vi "Maint_Glue_Wind.vi"(0 "VISA Refnum in":refnum<visa-resource-name>, 7 "VISA Refnum in 2":refnum<visa-resource-name>, 11 "error in (no error)":errorcluster) -> (4 "VISA Refnum out":refnum<visa-resource-name>, 8 "VISA Refnum out 2":refnum<visa-resource-name>, 15 "error out":errorcluster)   [LabVIEW 2016]
panel:
  in  "Home Button":bool
  in  "Down Button 2":bool
  in  "Up Button":bool
  in  "error in (no error) 2":errorcluster
  out "error out 2":errorcluster
  in  "Wind Forward":bool
  in  "Wind Reverse":bool
  in  "Glue Down Button":bool
  in  "GLUE UP":bool
  in  "EXIT":bool
  # "GLUE MOTOR"
  # "WIND MOTOR"
  # "STEPPER MOTOR"
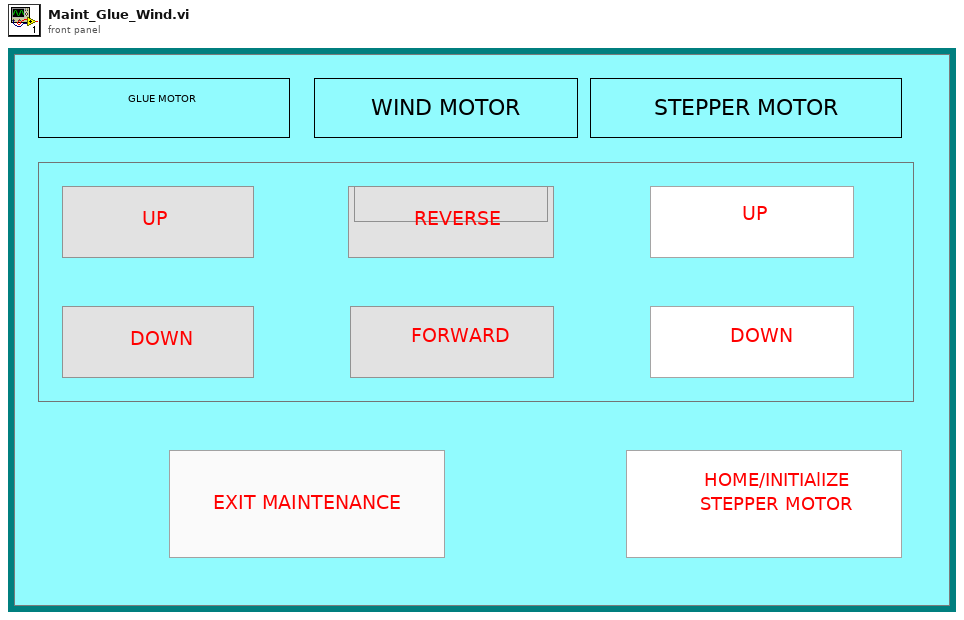
[diagram p1: front panel]
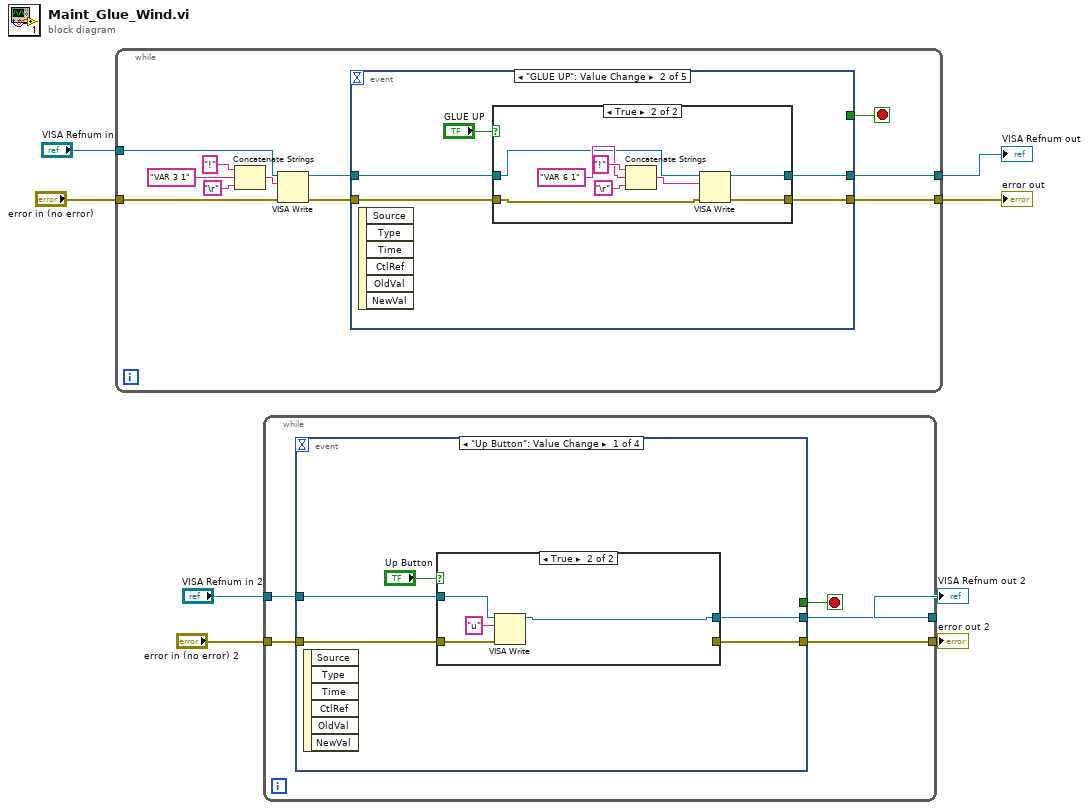
[diagram p0: block diagram]
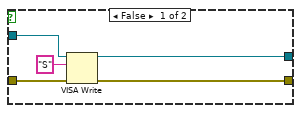
[diagram p2: hidden frame]
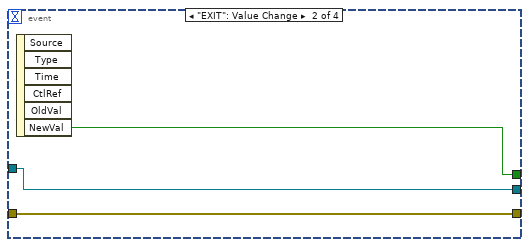
[diagram p3: hidden frame]
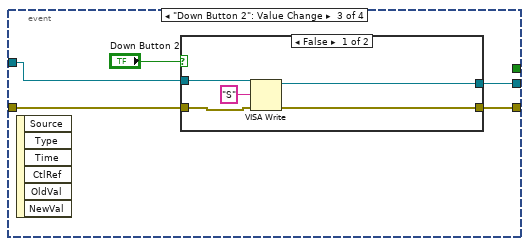
[diagram p4: hidden frame]
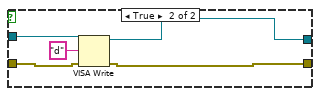
[diagram p5: hidden frame]
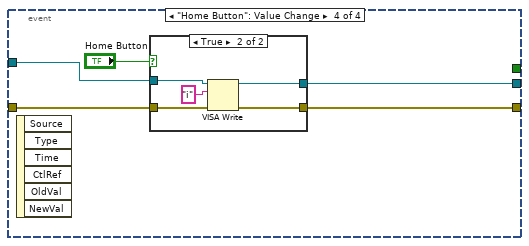
[diagram p6: hidden frame]
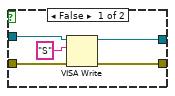
[diagram p7: hidden frame]
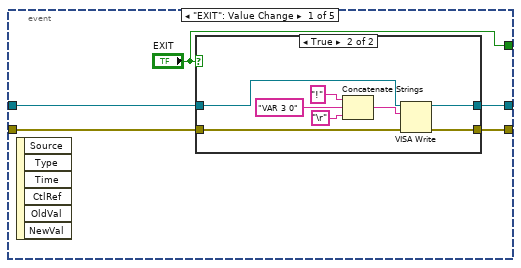
[diagram p8: hidden frame]
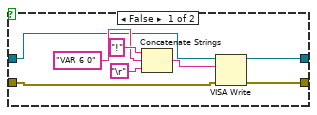
[diagram p10: hidden frame]
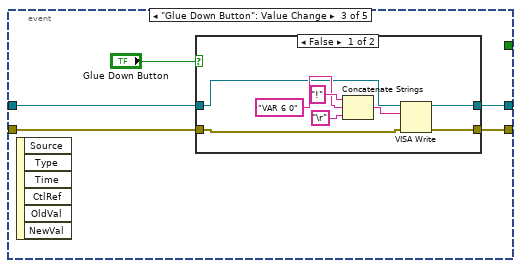
[diagram p11: hidden frame]
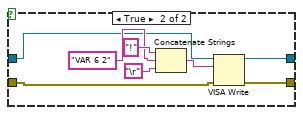
[diagram p12: hidden frame]
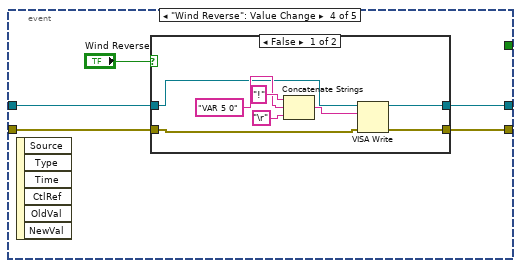
[diagram p13: hidden frame]
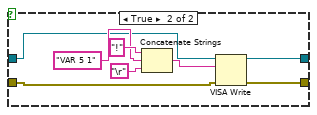
[diagram p14: hidden frame]
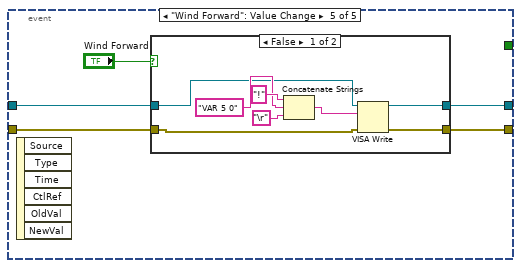
[diagram p15: hidden frame]
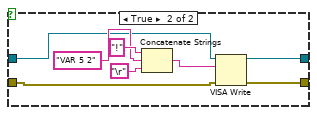
[diagram p16: hidden frame]
diagram:
  n1 = while {
    tunnel: "VISA Refnum in" -> [w12]
    tunnel: "error in (no error)" -> [w11]
    tunnel: [w10] -> w7
    tunnel: [w9] -> w8
    stop <- w13 stop-if-true
    n2 = Concatenate Strings("!" ("string to write 2"), "VAR 3 1" ("string"), "\r") -> (w17:string)
    n3 = VISA Write(VISA resource name=w12, write buffer=w17, error in (no error)=w11) -> (VISA resource name out=w15:refnum<visa-resource-name>, error out=w14:errorcluster)  [unwired: 1 out]
    n4 = event shown="[1] \"GLUE UP\": Value Change" {
      selector: _ -> [_ _ _ _ _]
      dyn-events: _ -> [_ _ _ _ _]
      timeout: _ -> [_ _ _ _ _]
      tunnel: [w20 w34 w55 w77 w97] -> w10
      tunnel: [w21 w33 w54 w76 w96] -> w9
      tunnel: w15 -> [w23 w36 w57 w79 w99]
      tunnel: w14 -> [w22 w35 w56 w78 w98]
      tunnel: ["EXIT" _ _ _ _] -> w13
      event "EXIT": Value Change {
        n5 = event-data() -> ()  [unwired: 1 in, 6 out]
        n6 = case shown="True" "EXIT" {
          tunnel: w23 -> [_ w32]
          tunnel: w22 -> [_ w31]
          tunnel: [_ w26] -> w21
          tunnel: [_ w25] -> w20
          frame False {
          }
          frame True {
            n7 = Concatenate Strings("!" ("string to write 2"), "VAR 3 0" ("string"), "\r") -> (w27:string)
            n8 = VISA Write(VISA resource name=w32, write buffer=w27, error in (no error)=w31) -> (VISA resource name out=w25:refnum<visa-resource-name>, error out=w26:errorcluster)  [unwired: 1 out]
          }
        }
      }
      event "GLUE UP": Value Change {
        n9 = event-data() -> ()  [unwired: 1 in, 6 out]
        n10 = case shown="True" "GLUE UP" {
          tunnel: w36 -> [w42 w49]
          tunnel: w35 -> [w41 w48]
          tunnel: [w40 w47] -> w34
          tunnel: [w39 w46] -> w33
          frame False {
            n11 = Concatenate Strings("!" ("string to write 2"), "VAR 6 0" ("string"), "\r") -> (w43:string)
            n12 = VISA Write(VISA resource name=w42, write buffer=w43, error in (no error)=w41) -> (VISA resource name out=w40:refnum<visa-resource-name>, error out=w39:errorcluster)  [unwired: 1 out]
          }
          frame True {
            n13 = Concatenate Strings("!" ("string to write 2"), "VAR 6 1" ("string"), "\r") -> (w51:string)
            n14 = VISA Write(VISA resource name=w49, write buffer=w51, error in (no error)=w48) -> (VISA resource name out=w47:refnum<visa-resource-name>, error out=w46:errorcluster)  [unwired: 1 out]
          }
        }
      }
      event "Glue Down Button": Value Change {
        n15 = event-data() -> ()  [unwired: 1 in, 6 out]
        n16 = case shown="False" "Glue Down Button" {
          tunnel: w57 -> [w62 w70]
          tunnel: w56 -> [w61 w69]
          tunnel: [w60 w68] -> w55
          tunnel: [w59 w67] -> w54
          frame False {
            n17 = Concatenate Strings("!" ("string to write 2"), "VAR 6 0" ("string"), "\r") -> (w64:string)
            n18 = VISA Write(VISA resource name=w62, write buffer=w64, error in (no error)=w61) -> (VISA resource name out=w60:refnum<visa-resource-name>, error out=w59:errorcluster)  [unwired: 1 out]
          }
          frame True {
            n19 = Concatenate Strings("!" ("string to write 2"), "VAR 6 2" ("string"), "\r") -> (w72:string)
            n20 = VISA Write(VISA resource name=w70, write buffer=w72, error in (no error)=w69) -> (VISA resource name out=w68:refnum<visa-resource-name>, error out=w67:errorcluster)  [unwired: 1 out]
          }
        }
      }
      event "Wind Reverse": Value Change {
        n21 = event-data() -> ()  [unwired: 1 in, 6 out]
        n22 = case shown="False" "Wind Reverse" {
          tunnel: w79 -> [w83 w91]
          tunnel: w78 -> [w82 w90]
          tunnel: [w80 w89] -> w77
          tunnel: [w81 w88] -> w76
          frame False {
            n23 = Concatenate Strings("!" ("string to write 2"), "VAR 5 0" ("string"), "\r") -> (w85:string)
            n24 = VISA Write(VISA resource name=w83, write buffer=w85, error in (no error)=w82) -> (VISA resource name out=w80:refnum<visa-resource-name>, error out=w81:errorcluster)  [unwired: 1 out]
          }
          frame True {
            n25 = Concatenate Strings("!" ("string to write 2"), "VAR 5 1" ("string"), "\r") -> (w93:string)
            n26 = VISA Write(VISA resource name=w91, write buffer=w93, error in (no error)=w90) -> (VISA resource name out=w89:refnum<visa-resource-name>, error out=w88:errorcluster)  [unwired: 1 out]
          }
        }
      }
      event "Wind Forward": Value Change {
        n27 = event-data() -> ()  [unwired: 1 in, 6 out]
        n28 = case shown="False" "Wind Forward" {
          tunnel: w99 -> [w104 w112]
          tunnel: w98 -> [w103 w111]
          tunnel: [w102 w110] -> w97
          tunnel: [w101 w109] -> w96
          frame False {
            n29 = Concatenate Strings("!" ("string to write 2"), "VAR 5 0" ("string"), "\r") -> (w106:string)
            n30 = VISA Write(VISA resource name=w104, write buffer=w106, error in (no error)=w103) -> (VISA resource name out=w102:refnum<visa-resource-name>, error out=w101:errorcluster)  [unwired: 1 out]
          }
          frame True {
            n31 = Concatenate Strings("!" ("string to write 2"), "VAR 5 2" ("string"), "\r") -> (w114:string)
            n32 = VISA Write(VISA resource name=w112, write buffer=w114, error in (no error)=w111) -> (VISA resource name out=w110:refnum<visa-resource-name>, error out=w109:errorcluster)  [unwired: 1 out]
          }
        }
      }
    }
  }
  "error out" <- w8
  "VISA Refnum out" <- w7
  n33 = while {
    tunnel: "VISA Refnum in 2" -> [w119]
    tunnel: [w121] -> w3
    tunnel: "error in (no error) 2" -> [w118]
    tunnel: [w120] -> w4
    stop <- w117 stop-if-true
    n34 = event shown="[0] \"Up Button\": Value Change" {
      selector: _ -> [_ _ _ _]
      dyn-events: _ -> [_ _ _ _]
      timeout: _ -> [_ _ _ _]
      tunnel: [w124 w137 w141 w155] -> w121
      tunnel: [w123 w136 w140 w154] -> w120
      tunnel: w119 -> [w126 w137 w143 w157]
      tunnel: w118 -> [w125 w136 w142 w156]
      tunnel: [_ w138 _ _] -> w117
      event "Up Button": Value Change {
        n35 = event-data() -> ()  [unwired: 1 in, 6 out]
        n36 = case shown="True" "Up Button" {
          tunnel: w126 -> [w130 w135]
          tunnel: w125 -> [w129 w134]
          tunnel: [w128 w132] -> w124
          tunnel: [w127 _] -> w123
          frame False {
            n37 = VISA Write(VISA resource name=w130, write buffer="S", error in (no error)=w129) -> (VISA resource name out=w128:refnum<visa-resource-name>, error out=w127:errorcluster)  [unwired: 1 out]
          }
          frame True {
            n38 = VISA Write(VISA resource name=w135, write buffer="u", error in (no error)=w134) -> (VISA resource name out=w132:refnum<visa-resource-name>)  [unwired: 2 out]
          }
        }
      }
      event "EXIT": Value Change {
        n39 = event-data() -> ("NewVal"=w138:bool)  [unwired: 1 in, 5 out]
      }
      event "Down Button 2": Value Change {
        n40 = event-data() -> ()  [unwired: 1 in, 6 out]
        n41 = case shown="False" "Down Button 2" {
          tunnel: w143 -> [w147 w153]
          tunnel: w142 -> [w146 w152]
          tunnel: [w145 w150] -> w141
          tunnel: [w144 w149] -> w140
          frame False {
            n42 = VISA Write(VISA resource name=w147, write buffer="S", error in (no error)=w146) -> (VISA resource name out=w145:refnum<visa-resource-name>, error out=w144:errorcluster)  [unwired: 1 out]
          }
          frame True {
            n43 = VISA Write(VISA resource name=w153, write buffer="d", error in (no error)=w152) -> (VISA resource name out=w150:refnum<visa-resource-name>, error out=w149:errorcluster)  [unwired: 1 out]
          }
        }
      }
      event "Home Button": Value Change {
        n44 = event-data() -> ()  [unwired: 1 in, 6 out]
        n45 = case shown="True" "Home Button" {
          tunnel: w157 -> [w162 w168]
          tunnel: w156 -> [w161 w167]
          tunnel: [w160 w166] -> w155
          tunnel: [w159 w165] -> w154
          frame False {
            n46 = VISA Write(VISA resource name=w162, write buffer="S", error in (no error)=w161) -> (VISA resource name out=w160:refnum<visa-resource-name>, error out=w159:errorcluster)  [unwired: 1 out]
          }
          frame True {
            n47 = VISA Write(VISA resource name=w168, write buffer="i", error in (no error)=w167) -> (VISA resource name out=w166:refnum<visa-resource-name>, error out=w165:errorcluster)  [unwired: 1 out]
          }
        }
      }
    }
  }
  "error out 2" <- w4
  "VISA Refnum out 2" <- w3
